vi "UnMarshall.vi"(7 "Type":variant, 8 "error in (no error)":errorcluster, 10 "String":string, 11 "Serializer in":refnum<class "Serializer.lvclass">) -> (0 "error out":errorcluster, 2 "Variant":variant, 3 "Serializer out":refnum<class "Serializer.lvclass">)   [LabVIEW 2013, in "SMOConfig.lvlib" / "Serializer.lvclass"]
uses:
  Serializer.lvclass
  <vilib>/addons/_JKI.lib/Serialization/JSON/JKI JSON Serialization.lvlib
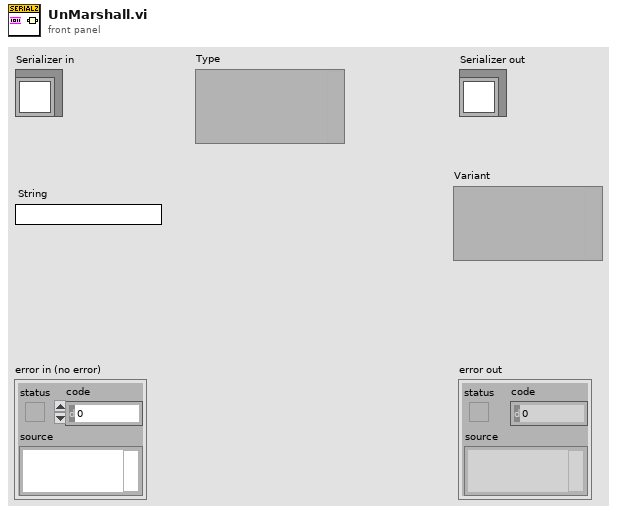
[diagram p1: front panel]
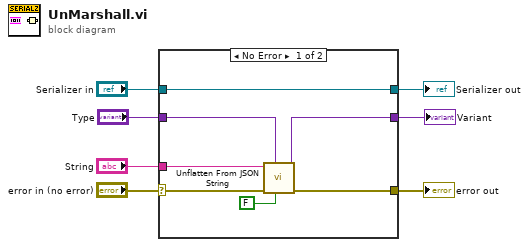
[diagram p0: block diagram]
diagram:
  n1 = case shown="No Error" "error in (no error)" {
    selector: "error in (no error)" -> [w12 w16]
    tunnel: [w10 w16] -> w6
    tunnel: [w14 w15] -> w4
    tunnel: "Serializer in" -> [w14 w15]
    tunnel: [w9 _] -> w3
    tunnel: "Type" -> [w11 _]
    tunnel: "String" -> [w13 _]
    frame No Error {
      n2 = call <vilib>:"Unflatten From JSON String.vi"("Nulls as Defaults (F)"=FALSE, "Type and Defaults"=w11, "error in (no error)"=w12, "JSON String"=w13) -> ("error out"=w10:errorcluster, "Variant"=w9:variant)  [unwired: 6 in]
    }
    frame Error {
    }
  }
  "error out" <- w6
  "Serializer out" <- w4
  "Variant" <- w3
